vi "Dlg-Add-Operation.vi"(8 "error in (no error)":errorcluster, 11 "Operations in":refnum<class "Operations.lvclass">) -> (0 "error out":errorcluster, 2 "Canceled":bool, 3 "Operations out":refnum<class "Operations.lvclass">)   [LabVIEW 2012]
uses:
  Operation/Operation Type Enum.ctl
  controls/Currencies.ctl
  Operations.lvclass
  Operation/Operation.lvclass
  Operation/Operation Parameters.ctl
  Operation/Operation.lvclass/Operation.ctl
panel:
  in  "Currency":T1
  in  "Montant":dbl
  in  "Type d'opération":T2
  in  "Add":bool
  in  "Date":timestamp format="%<%X\n%x>T"
  in  "Commentaires":string
  in  "Cancel Button":bool
  in  "Help":bool
  # "Nouveau Portefeuille"
  # "Ajouter une Opération"
  # "Opération"
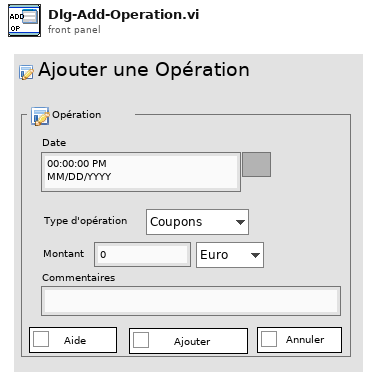
[diagram p1: front panel]
types:
  T1 = typedef "Currencies.ctl" = enum16{"Euro", "Dollar", "Yen", "RIM", "CHF"}
  T2 = typedef "Operation Type Enum.ctl" = enum16{"Coupons", "Dépot", "Retrait", "Intérêts", "Taxe"}
  T3 = typedef "Operation Parameters.ctl" = cluster{"Date":timestamp, "Operation Type":T2, "Amount":dbl, "Comment":string, "Currency":T1}
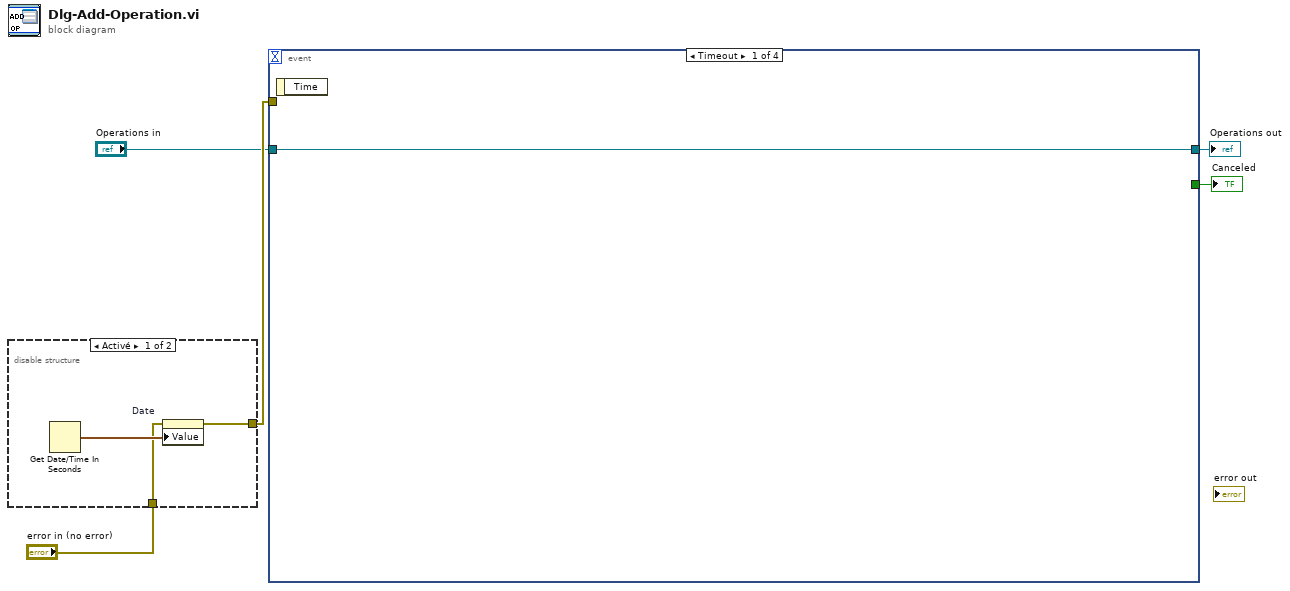
[diagram p0: block diagram]
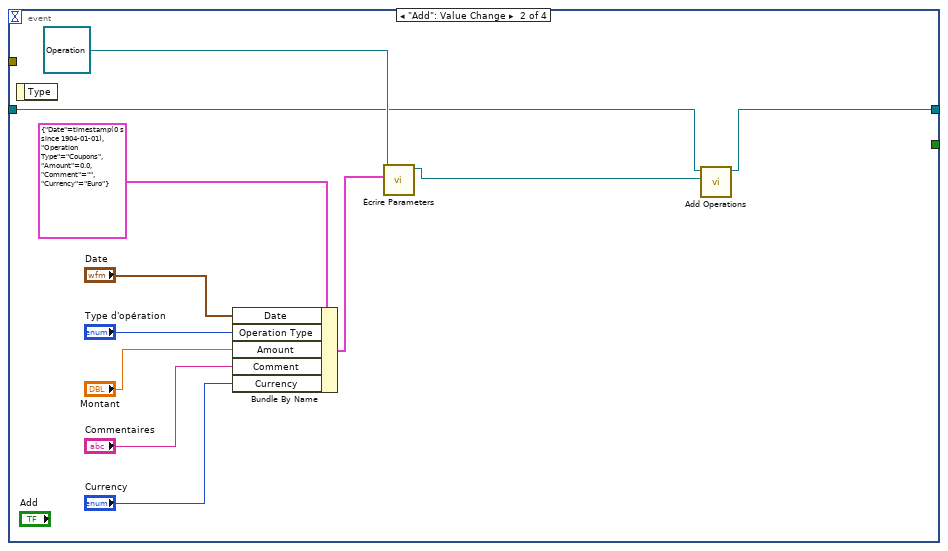
[diagram p3: hidden frame]
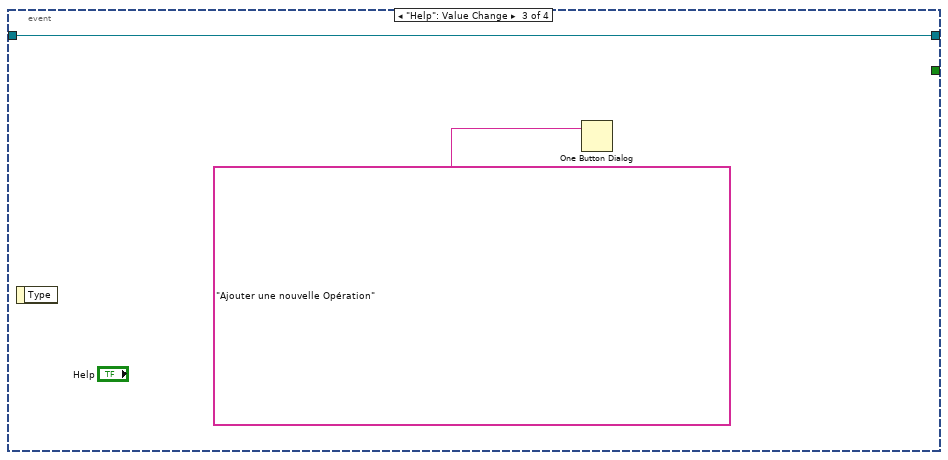
[diagram p4: hidden frame]
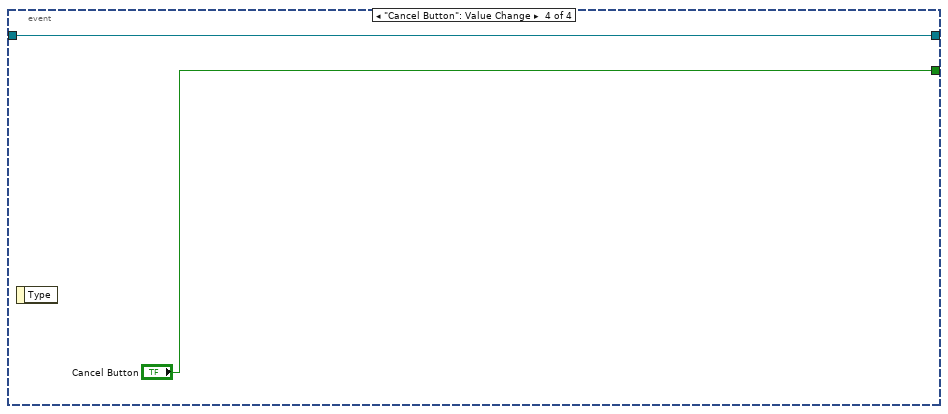
[diagram p5: hidden frame]
diagram:
  n1 = disable-structure shown="Activé" {
    disable-tunnel: [w7 _] -> w5
    disable-tunnel: "error in (no error)" -> [w6 _]
    frame Enabled {
      n2 = Get Date/Time In Seconds() -> (seconds since 1Jan1904=w8:timestamp)
      n3 = property on="Date" class="TempsAbs (strict)"(error in=w6, "Value"=w8) -> (error out=w7:errorcluster)  [unwired: 1 in, 1 out]
    }
    frame Disabled {
    }
  }
  n4 = event shown="[0] Timeout" {
    selector: _ -> [_ _ _ _]
    dyn-events: _ -> [_ _ _ _]
    timeout: _ -> [_ _ _ _]
    tunnel: w5 -> [_ _ _ _]
    tunnel: [_ _ _ "Cancel Button"] -> w3
    tunnel: "Operations in" -> [w9 w11 w21 w23]
    tunnel: [w9 w10 w21 w23] -> w1
    event Timeout {
      n5 = event-data() -> ()  [unwired: 1 in, 1 out]
    }
    event "Add": Value Change {
      n6 = event-data() -> ()  [unwired: 1 in, 1 out]
      n7 = Bundle By Name(cluster=T3 {"Date"=timestamp(0 s since 1904-01-01), "Operation Type"=enum."Coupons", "Amount"=0.0, "Comment"="", "Currency"=enum."Euro"} ("Parameters"), "Date"="Date", "Operation Type"="Type d'opération", "Amount"="Montant", "Comment"="Commentaires", "Currency"="Currency") -> (w13:T3)
      n8 = call "Écrire Parameters.vi"("Parameters"=w13, "Operation en entrée"=refnum<class "Operation.lvclass"> refnum ("Operation.lvclass")) -> ("Operation en sortie"=w12:refnum<class "Operation.lvclass">)  [unwired: 9 in]
      n9 = call "Add Operations.vi"("Added Operation"=w12, "Operations en entrée"=w11) -> ("Operations en sortie"=w10:refnum<class "Operations.lvclass">)  [unwired: 7 in, 2 out]
    }
    event "Help": Value Change {
      n10 = event-data() -> ()  [unwired: 1 in, 1 out]
      n11 = One Button Dialog(message="Ajouter une nouvelle Opération") -> ()  [unwired: 1 in, 1 out]
    }
    event "Cancel Button": Value Change {
      n12 = event-data() -> ()  [unwired: 1 in, 1 out]
    }
  }
  "Canceled" <- w3
  "Operations out" <- w1
